vi "Wait for Laser.vi"(8 "error in (no error)":errorcluster, 10 "Desired State":T1, 11 "Recipe Process in":refnum<class "Recipe Process.lvclass">) -> (0 "error out":errorcluster, 3 "Recipe Process out":refnum<class "Recipe Process.lvclass">)   [LabVIEW 2022 SP3, in "Recipe Process.lvlib" / "Recipe Process.lvclass"]
uses:
  Recipe Process.lvclass
  Recipe Process.lvclass/Recipe Process.ctl
  Laser/Laser Controller api/Laser API.lvclass
  XY Stage/Process Actor/Process Framework/Process State Data/Process State Data.lvclass
  Laser/Laser State Data/Laser State.ctl
  Laser/Laser State Data/Laser State Data.lvclass
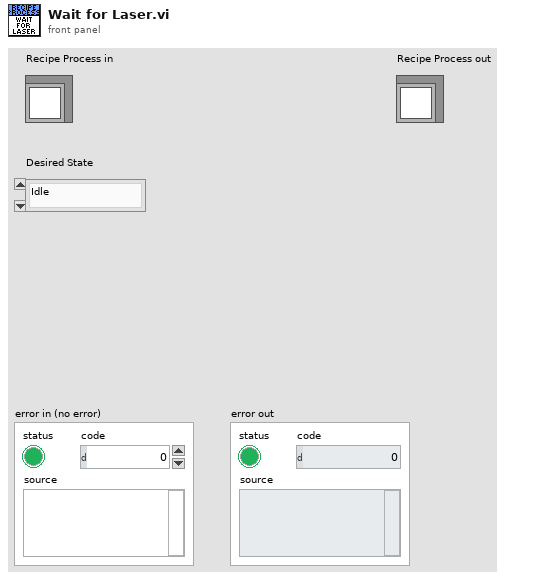
[diagram p1: front panel]
types:
  T1 = typedef "Laser State Data.lvclass/Laser State.ctl" = enum16{"Idle", "Warming", "Ready", "Firing"}
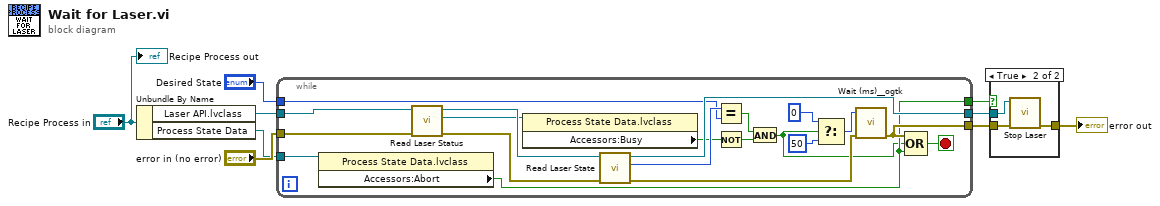
[diagram p0: block diagram]
diagram:
  n1 = Unbundle By Name("Recipe Process in") -> ("Laser API.lvclass"=w6:refnum<class "Laser API.lvclass">, "Process State Data"=w7:refnum<data-value>)
  n2 = while {
    tunnel: w6 -> [w16]
    tunnel: "error in (no error)" -> [w28]
    tunnel: w7 -> [w21]
    tunnel: [w20] -> w3
    tunnel: [w19] -> w4
    tunnel: [w18] -> w5
    tunnel: "Desired State" -> [w10]
    stop <- w23 stop-if-true
    n3 = property class="Process State Data.lvclass"(reference=w21) -> ("Accessors:Abort"=w18:bool)  [unwired: 1 in, 2 out]
    n4 = call-dynamic "Read Laser Status.vi"("error in (no error)"=w28, "Get Laser Status in"=w16) -> ("error out"=w17:errorcluster, "Process State Data"=w14:refnum<data-value>, "Get Laser Status out"=w15:refnum<class "Laser API.lvclass">)  [unwired: 7 in]
    n5 = property class="Process State Data.lvclass"(reference=w14) -> ("Accessors:Busy"=w13:bool)  [unwired: 1 in, 2 out]
    n6 = call-dynamic "Read Laser State.vi"("error in (no error)"=w17, "Get Laser Status in"=w15) -> ("error out"=w24:errorcluster, "Laser State"=w29:T1, "Get Laser Status out"=w19:refnum<class "Laser API.lvclass">)  [unwired: 7 in]
    n7 = Equal?(x=w29, y=w10) -> (x = y?=w22:bool)
    n8 = Not(x=w13) -> (.not. x?=w11:bool)
    n9 = And(x=w22, y=w11) -> (x .and. y?=w12:bool)
    n10 = Select(t=u32 0 ("milliseconds to wait"), s=w12, f=u32 50) -> (s? t:f=w25:u32)
    n11 = call <userlib>:"Wait (ms)__ogtk.vi"("error in (no error)"=w24, "milliseconds to wait"=w25) -> ("error out"=w20:errorcluster)  [unwired: 8 in, 1 out]
    n12 = Compound Arithmetic op=OR(w20, w12, w18) -> (w23:bool)
  }
  n13 = case shown="True" w5 {
    tunnel: w4 -> [_ w33]
    tunnel: w3 -> [w30 w32]
    tunnel: [w30 w31] -> w2
    frame False {
    }
    frame True {
      n14 = call-dynamic "Stop Laser.vi"("error in (no error)"=w32, "Laser API in"=w33) -> ("error out"=w31:errorcluster)  [unwired: 8 in, 1 out]
    }
  }
  "error out" <- w2
  "Recipe Process out" <- "Recipe Process in"
